vi "front_panel_change_subvi.vi"(0 "index":i32, 1 "Boolean":bool, 5 "locked reference":refnum<vi>, 7 "PD reference":refnum<vi>, 9 "setpoint voltage reference":refnum<vi>, 12 "PD":dbl[](array[numeric]), 13 "locked":bool[](array[boolean]), 14 "setpoint voltage":dbl[](array[numeric])) -> (4 "photodiode":dbl(graph), 6 "setpoint voltage (0V - 2V)":dbl(graph), 10 "locked":bool[](array[boolean])=[TRUE])   [LabVIEW 2015]
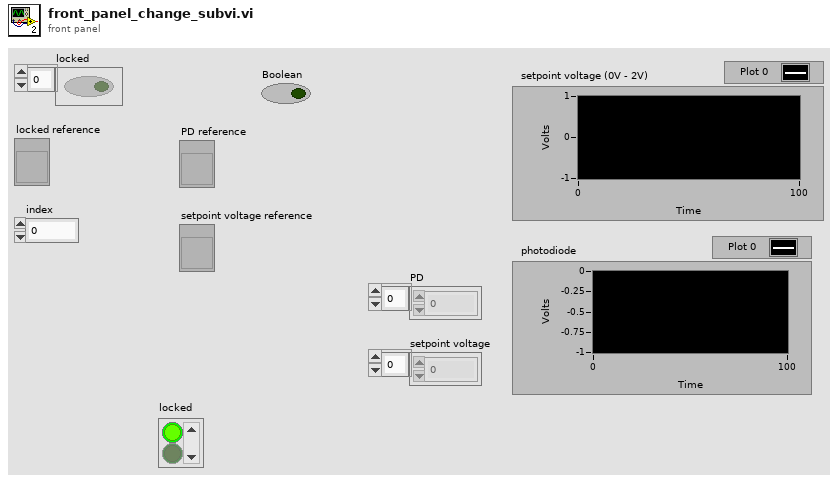
[diagram p1: front panel]
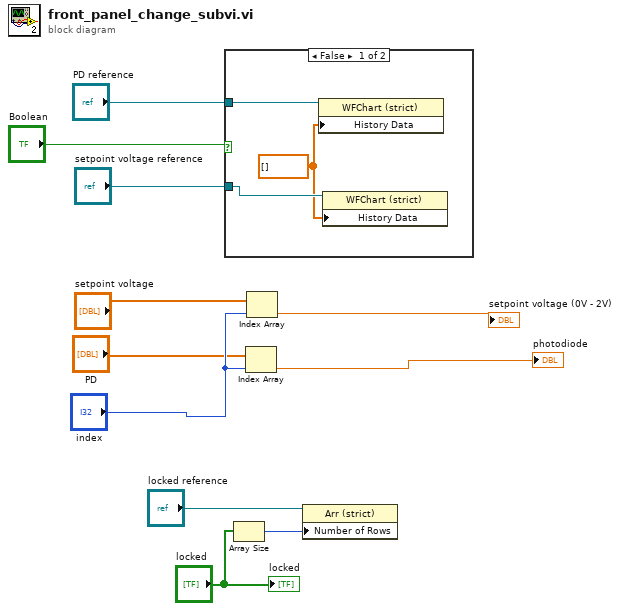
[diagram p0: block diagram]
diagram:
  n1 = case shown="False" "Boolean" {
    tunnel: "PD reference" -> [w14 _]
    tunnel: "setpoint voltage reference" -> [w13 _]
    frame False {
      w12 = dbl[] [] ("History Data")
      n2 = property on="Property Node" class="WFChart (strict)"(reference=w14, "History Data"=w12) -> ()  [unwired: 1 in, 2 out]
      n3 = property on="Property Node" class="WFChart (strict)"(reference=w13, "History Data"=w12) -> ()  [unwired: 1 in, 2 out]
    }
    frame True {
    }
  }
  n4 = Array Size(array="locked") -> (size(s)=w11:i32)
  n5 = Index Array(array="PD", index="index") -> (element=→"photodiode":dbl)
  n6 = Index Array(array="setpoint voltage", index="index") -> (element=→"setpoint voltage (0V - 2V)":dbl)
  n7 = property on="Property Node" class="Arr (strict)"(reference="locked reference", "Number of Rows"=w11) -> ()  [unwired: 1 in, 2 out]
  "locked" <- "locked"
